vi "Read Record Data.vi"(8 "Error In (no error)":errorcluster, 11 "Expenses Tracker Saving Goal In":refnum<class "Expenses Tracker Saving.lvclass">) -> (0 "Error Out":errorcluster, 2 "Record":variant, 3 "Expenses Tracker Saving Goal Out":refnum<class "Expenses Tracker Saving.lvclass">)   [LabVIEW 2023, in "Expenses Tracker Saving.lvclass"]
uses:
  Expenses Tracker Saving.lvclass
  Expenses Tracker Saving.lvclass/Expenses Tracker Saving.ctl
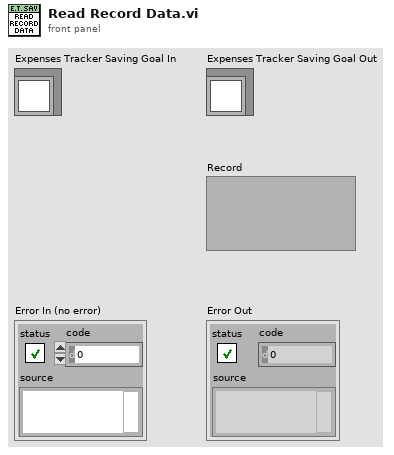
[diagram p1: front panel]
types:
  T1 = typedef "Expenses Tracker Record.lvclass/Saving.ctl" = cluster{"ID":u32, "Saving_goal":u32, "Value":dbl, "Date_of_entry":timestamp, "Description":string}
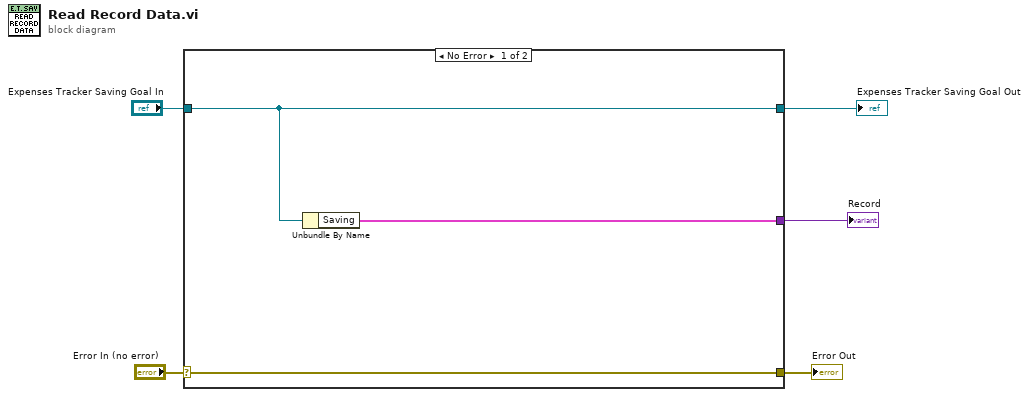
[diagram p0: block diagram]
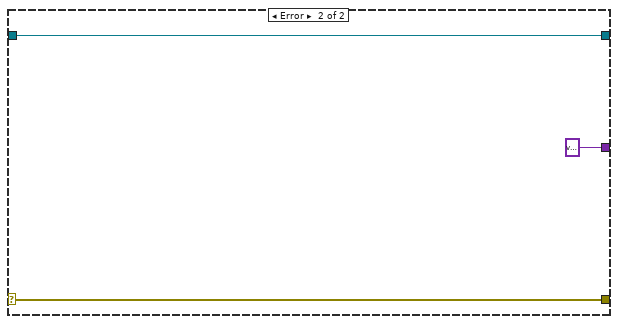
[diagram p2: hidden frame]
diagram:
  n1 = case shown="No Error" "Error In (no error)" {
    selector: "Error In (no error)" -> [w8 w11]
    tunnel: [w8 w11] -> w2
    tunnel: [w7 w10] -> w5
    tunnel: "Expenses Tracker Saving Goal In" -> [w7 w10]
    tunnel: [w6 variant] -> w1
    frame No Error {
      n2 = Unbundle By Name(w7) -> ("Saving"=w6:T1)
    }
    frame Error {
    }
  }
  "Error Out" <- w2
  "Expenses Tracker Saving Goal Out" <- w5
  "Record" <- w1
